vi "TrackingComm.vi"(3 "server address":string="192.168.0.101") -> (0 "error out":errorcluster, 1 "connected to server?":bool)   [LabVIEW 2017]
uses:
  libowlsock.dll
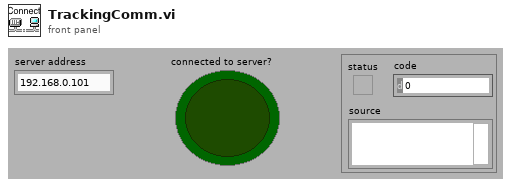
[diagram p1: front panel]
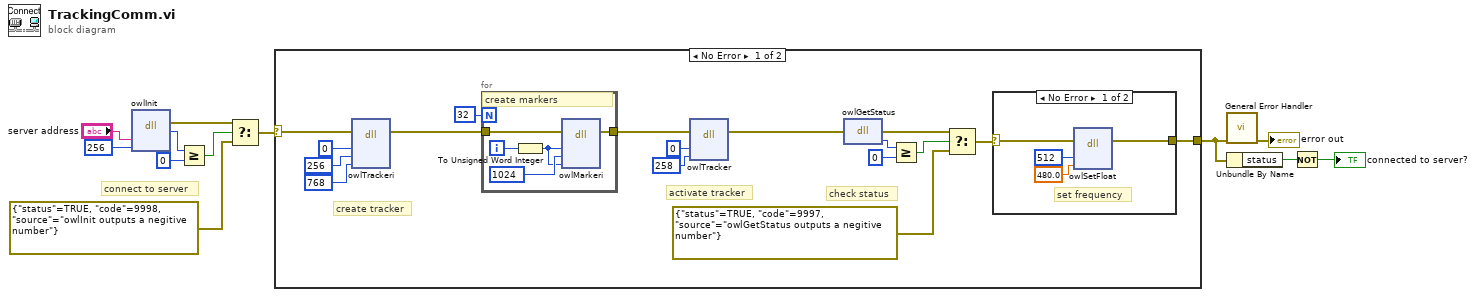
[diagram p0: block diagram]
diagram:
  # "connect to server"
  n1 = dll-call lib="libowlsock.dll" fn="owlInit"("server"="server address", "flags"=u16 256) -> (error out=w6:errorcluster, "return type"=w10:i16)  [unwired: 5 in, 1 out]
  n2 = Greater Or Equal?(x=w10, y=i16 0) -> (x >= y?=w7:bool)
  n3 = Select(t=w6, s=w7, f=errorcluster {"status"=TRUE, "code"=9998, "source"="owlInit outputs a negitive number"} ("error out")) -> (s? t:f=w5:errorcluster)
  n4 = case shown="No Error" w5 {
    selector: w5 -> [w28 w40]
    tunnel: [w29 w40] -> w3
    frame No Error {
      # "activate tracker"
      # "create tracker"
      # "check status"
      n5 = dll-call lib="libowlsock.dll" fn="owlTrackeri"(error in=w28, "tracker"=u16 0 ("y"), "pname"=u16 256 ("flags"), "param"=u16 768 ("flags")) -> (error out=w19:errorcluster)  [unwired: 5 in, 2 out]
      n6 = for {
        N: 32 -> [_]
        tunnel: w19 -> [w32]
        tunnel: [w31] -> w21
        i -> [w34]
        # "create markers"
        n7 = To Unsigned Word Integer(number=w34) -> (unsigned 16bit integer=w30:u16)
        n8 = dll-call lib="libowlsock.dll" fn="owlMarkeri"(error in=w32, "marker"=w30, "pname"=u16 1024 ("flags"), "param"=w30) -> (error out=w31:errorcluster)  [unwired: 3 in, 4 out]
      }
      n9 = dll-call lib="libowlsock.dll" fn="owlTracker"(error in=w21, "tracker"=u16 0, "pname"=u16 258 ("flags")) -> (error out=w27:errorcluster)  [unwired: 4 in, 2 out]
      n10 = dll-call lib="libowlsock.dll" fn="owlGetStatus"(error in=w27) -> (error out=w15:errorcluster, "return type"=w25:u16)  [unwired: 2 in, 1 out]
      n11 = Greater Or Equal?(x=w25, y=u16 0) -> (x >= y?=w16:bool)
      n12 = Select(t=w15, s=w16, f=errorcluster {"status"=TRUE, "code"=9997, "source"="owlGetStatus outputs a negitive number"} ("error out")) -> (s? t:f=w14:errorcluster)
      n13 = case shown="No Error" w14 {
        selector: w14 -> [w36 w39]
        tunnel: [w35 w39] -> w29
        frame No Error {
          # "set frequency"
          n14 = dll-call lib="libowlsock.dll" fn="owlSetFloat"(error in=w36, "pname"=u16 512, "param"=sgl 480.0) -> (error out=w35:errorcluster)  [unwired: 4 in, 2 out]
        }
        frame Error {
        }
      }
    }
    frame Error {
    }
  }
  n15 = call <vilib>:"General Error Handler.vi"("error in (no error)"=w3) -> ("error out"=→"error out":errorcluster)  [unwired: 3 in, 11 out]
  n16 = Unbundle By Name(w3) -> ("status"=w2:bool)
  n17 = Not(x=w2) -> (.not. x?=→"connected to server?":bool)
